vi "Set Display State.vi"(0 "Picture Array Refnum":refnum<vi>, 1 "Facade Vi Refnum":refnum<vi>, 2 "Container Refnum":refnum<vi>, 3 "Display State In":T1={"Buttons Displayed"=0, "Button States"=[], "Button Size"=0, "Button Style"=enum."Classic", "Active Button"=0, "Force Regen?"=FALSE, "Tip String Ref"=refnum} caption="State", 4 "Display":picture[](array[picture])) -> (5 "State Out":T1={"Buttons Displayed"=0, "Button States"=[], "Button Size"=0, "Button Style"=enum."Classic", "Active Button"=0, "Force Regen?"=FALSE, "Tip String Ref"=refnum} caption="State", 6 "Images Out":picture[](array[picture]))   [LabVIEW 2012, in "Toolbar.xctl"]
doc: "Adjusts the facade array of pictures to have the appearance required to accommodate the display state of the toolbar (button sizes, number of buttons etc)."
uses:
  Toolbar.xctl
  Toolbar State.ctl
  Button_Class/Button.lvclass
  Button_Class/Type Defs/Button Style.ctl
panel:
  out "error out":errorcluster
  in  "error in (no error)":errorcluster
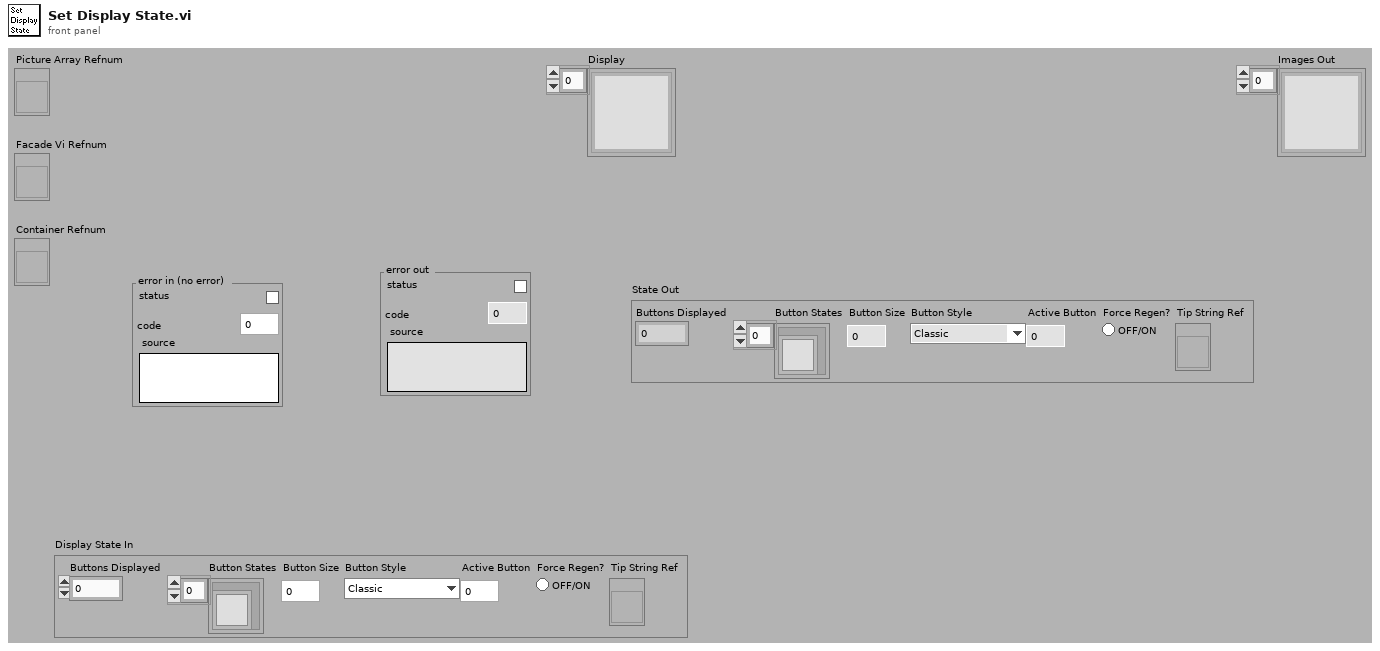
[diagram p1: front panel]
types:
  T1 = typedef "Toolbar.xctl/Toolbar State.ctl" = cluster{"Buttons Displayed":i32, "Button States":refnum<class "Button.lvclass">[], "Button Size":i32, "Button Style":T2, "Active Button":i32, "Force Regen?":bool, "Tip String Ref":refnum<vi>}
  T2 = typedef "Button.lvclass/Button Style.ctl" = enum16{"System", "Modern", "Classic", "Rounded", "Silver", "Ni Theme", "Metallic"}
  T3 = typedef "LVPositionTypeDef.ctl" = cluster{"Left":i32, "Top":i32}
  T4 = typedef "LVBoundsTypeDef.ctl" = cluster{"Width":u32, "Height":u32}
  T5 = typedef "LVRectTypeDef.ctl" = cluster{"Left":i16, "Top":i16, "Right":i16, "Bottom":i16}
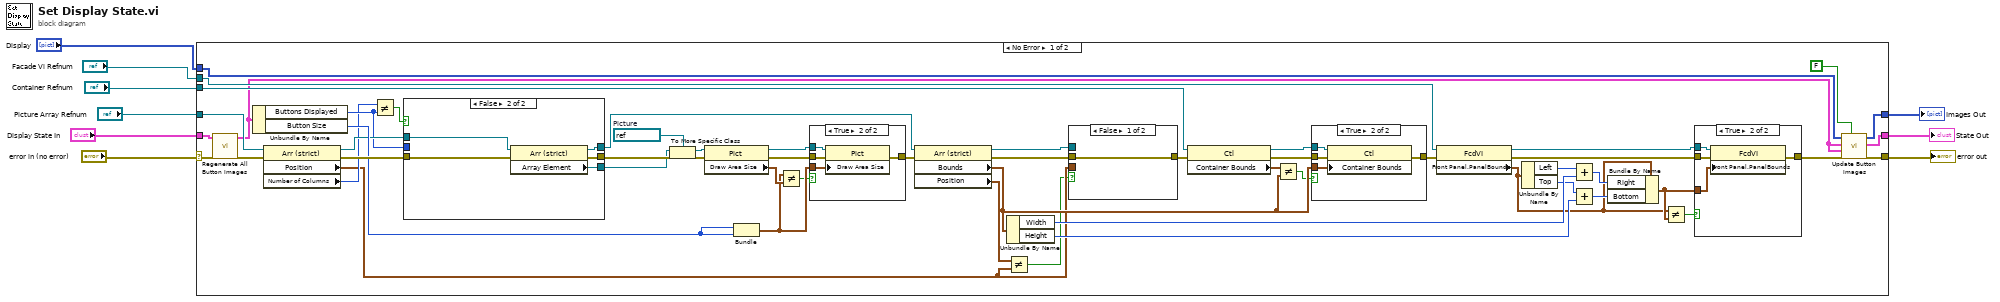
[diagram p0: block diagram]
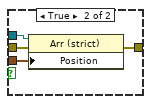
[diagram p2: hidden frame]
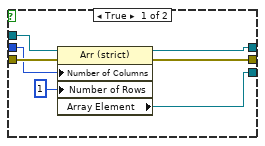
[diagram p4: hidden frame]
diagram:
  n1 = case shown="No Error" "error in (no error)" {
    selector: "error in (no error)" -> [w12 w96]
    tunnel: "Display State In" -> [w13 w97]
    tunnel: [w56 w97] -> w8
    tunnel: [w55 _] -> w7
    tunnel: "Display" -> [w54 _]
    tunnel: "Picture Array Refnum" -> [w49 _]
    tunnel: "Facade Vi Refnum" -> [w46 _]
    tunnel: "Container Refnum" -> [w32 _]
    tunnel: [w26 w96] -> w1
    frame No Error {
      w59 = refnum<vi> refnum  # Picture
      n2 = call "Regenerate All Button Images.vi"("error in (no error)"=w12, "Display State In in"=w13) -> ("error out"=w11:errorcluster, "Display State In out"=w10:T1)  [unwired: 8 in]
      n3 = Unbundle By Name(w10) -> ("Buttons Displayed"=w25:i32, "Button Size"=w62:i32)
      n4 = property on="Property Node" class="Arr (strict)"(reference=w49, error in=w11) -> (reference out=w48:refnum<vi>, error out=w63:errorcluster, "Position"=w15:T3, "Number of Columns"=w24:u32)
      n5 = Not Equal?(x=w24, y=w25) -> (x != y?=w23:bool)
      n6 = case shown="False" w23 {
        tunnel: w63 -> [w80 w85]
        tunnel: [w79 w84] -> w61
        tunnel: [w78 w83] -> w58
        tunnel: [w76 w82] -> w50
        tunnel: w48 -> [w75 w81]
        tunnel: w25 -> [w74 _]
        frame True {
          n7 = property on="Property Node" class="Arr (strict)"(reference=w75, error in=w80, "Number of Columns"=w74, "Number of Rows"=u32 1) -> (reference out=w76:refnum<vi>, error out=w79:errorcluster, "Array Element"=w78:refnum<vi>)
        }
        frame False {
          n8 = property on="Property Node" class="Arr (strict)"(reference=w81, error in=w85) -> (reference out=w82:refnum<vi>, error out=w84:errorcluster, "Array Element"=w83:refnum<vi>)
        }
      }
      n9 = To More Specific Class(target class=w59, reference=w58, error in=w61) -> (specific class reference=w60:refnum<vi>, error out=w21:errorcluster)
      n10 = property class="Pict"(reference=w60, error in=w21) -> (reference out=w22:refnum<vi>, error out=w20:errorcluster, "Draw Area Size"=w19:T4)
      n11 = Bundle("Button Size"=w62, "Button Size"=w62) -> (w18:cluster{"Button Size":i32, "Button Size":i32})  [unwired: 1 out]
      n12 = Not Equal?(x=w18, y=w19) -> (x != y?=w17:bool)
      n13 = case shown="True" w17 {
        tunnel: [w69 w73] -> w51
        tunnel: w22 -> [_ w72]
        tunnel: w20 -> [w69 w71]
        tunnel: w18 -> [_ w70]
        frame False {
        }
        frame True {
          n14 = property class="Pict"(reference=w72, error in=w71, "Draw Area Size"=w70) -> (error out=w73:errorcluster)  [unwired: 1 out]
        }
      }
      n15 = property on="Property Node" class="Arr (strict)"(reference=w50, error in=w51) -> (reference out=w53:refnum<vi>, error out=w52:errorcluster, "Bounds"=w29:T4, "Position"=w16:T3)
      n16 = Unbundle By Name(w29) -> ("Width"=w44:u32, "Height"=w42:u32)
      n17 = Not Equal?(x=w16, y=w15) -> (x != y?=w14:bool)
      n18 = case shown="False" w14 {
        tunnel: w53 -> [_ w68]
        tunnel: w52 -> [w64 w67]
        tunnel: [w64 w66] -> w34
        tunnel: w15 -> [_ w65]
        frame False {
        }
        frame True {
          n19 = property on="Property Node" class="Arr (strict)"(reference=w68, error in=w67, "Position"=w65) -> (error out=w66:errorcluster)  [unwired: 1 out]
        }
      }
      n20 = property class="Ctl"(reference=w32, error in=w34) -> (reference out=w31:refnum<vi>, error out=w33:errorcluster, "Container Bounds"=w30:T4)
      n21 = Not Equal?(x=w30, y=w29) -> (x != y?=w28:bool)
      n22 = case shown="True" w28 {
        tunnel: [w86 w90] -> w47
        tunnel: w33 -> [w86 w89]
        tunnel: w31 -> [_ w88]
        tunnel: w29 -> [_ w87]
        frame False {
        }
        frame True {
          n23 = property class="Ctl"(reference=w88, error in=w89, "Container Bounds"=w87) -> (error out=w90:errorcluster)  [unwired: 1 out]
        }
      }
      n24 = property class="FcdVI"(reference=w46, error in=w47) -> (reference out=w38:refnum<vi>, error out=w39:errorcluster, "Front Panel.PanelBounds"=w36:T5)
      n25 = Unbundle By Name(w36) -> ("Left"=w45:i16, "Top"=w43:i16)
      n26 = Add(x=w45, y=w44) -> (x+y=w41:u32)
      n27 = Add(x=w43, y=w42) -> (x+y=w40:u32)
      n28 = Bundle By Name(cluster=w36, "Right"=w41, "Bottom"=w40) -> (w37:T5)
      n29 = Not Equal?(x=w36, y=w37) -> (x != y?=w35:bool)
      n30 = case shown="True" w35 {
        tunnel: w39 -> [w91 w95]
        tunnel: w38 -> [_ w94]
        tunnel: w37 -> [_ w93]
        tunnel: [w91 w92] -> w27
        frame False {
        }
        frame True {
          n31 = property class="FcdVI"(reference=w94, error in=w95, "Front Panel.PanelBounds"=w93) -> (error out=w92:errorcluster)  [unwired: 1 out]
        }
      }
      n32 = call "Update Button Images.vi"("Force Regen"=FALSE, "error in (no error)"=w27, "Old State"=w10, "New State"=w10, "Images In"=w54) -> ("error out"=w26:errorcluster, "State Out"=w56:T1, "Images Out"=w55:picture[])  [unwired: 2 in, 2 out]
    }
    frame Error {
    }
  }
  "State Out" <- w8
  "Images Out" <- w7
  "error out" <- w1
